vi "Save_Destination_Type.vi"(8 "error in (no error)":errorcluster, 9 "index":string, 10 "buildObject":T1, 11 "absFolder in":refnum<class "absFolder.lvclass">) -> (0 "error out":errorcluster, 1 "index out":string, 2 "buildObject out":T1, 3 "absFolder out":refnum<class "absFolder.lvclass">)   [LabVIEW 2020, in "absFolder.lvclass"]
uses:
  <vilib>/AppBuilder/IB_Classes/Destination/absFolder/absFolder.lvclass
  <vilib>/AppBuilder/IB_Classes/Destination/absFolder/absFolder.lvclass/absFolder.ctl
  <resource>/Framework/Providers/API/ItemRef.ctl
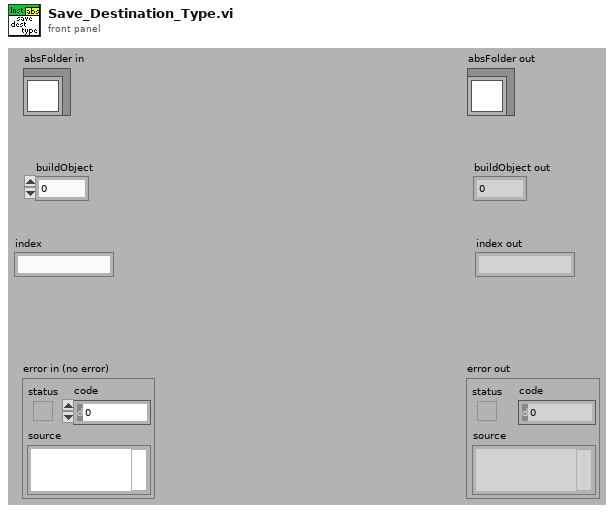
[diagram p1: front panel]
types:
  T1 = typedef "ItemRef.ctl" = u64
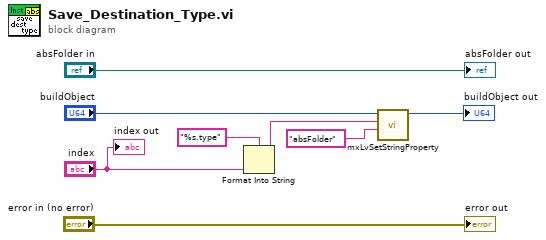
[diagram p0: block diagram]
diagram:
  n1 = Format Into String(format string="%s.type", "index") -> (resulting string=w7:string)  [unwired: 2 in, 1 out]
  n2 = call <resource>:"mxLvSetStringProperty.vi"("Value (\"\")"="absFolder" ("Value (\"\")"), "Tag"=w7, "Item"="buildObject") -> ("Item"=→"buildObject out":T1)  [unwired: 7 in, 1 out]
  "error out" <- "error in (no error)"
  "absFolder out" <- "absFolder in"
  "index out" <- "index"
